vi "DisposeCore.vi"(8 "error in (no error)":errorcluster, 11 "ProductA":refnum<class "ProductA.lvclass">) -> (0 "error out":errorcluster, 3 "ProductA":refnum<class "ProductA.lvclass">)   [LabVIEW 2020, in "FactoryMethod.lvlib" / "FactoryMethodLazyEvaluation.lvlib" / "ProductA.lvclass"]
uses:
  ProductA.lvclass
  Private/TypeDef/privateDataDVR.ctl
  Private/TypeDef/privateData.ctl
  ProductA.lvclass/ProductA.ctl
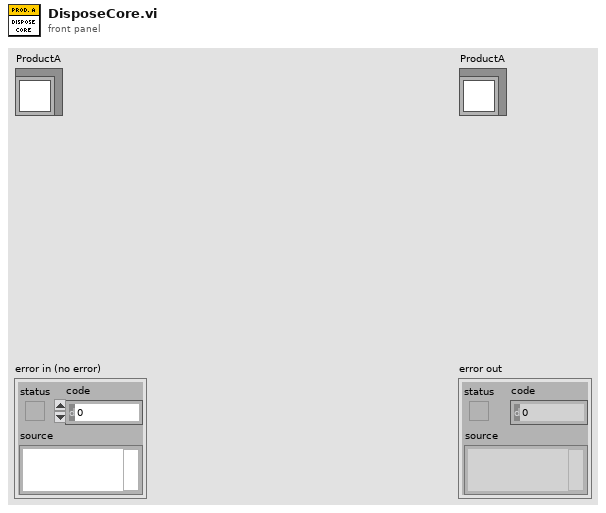
[diagram p1: front panel]
types:
  T1 = typedef "FactoryMethod.lvlib/FactoryMethodLazyEvaluation.lvlib/ProductA.lvclass/privateDataDVR.ctl" = refnum<data-value>
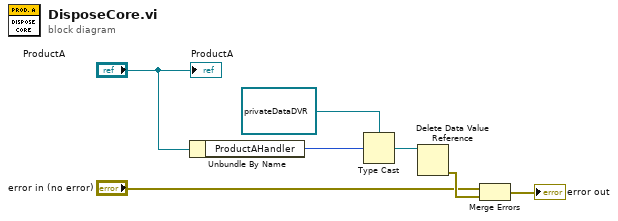
[diagram p0: block diagram]
diagram:
  n1 = Unbundle By Name("ProductA") -> ("ProductAHandler"=w7:u32)
  n2 = Type Cast(type=T1 refnum ("privateDataDVR"), x=w7) -> (*(type *) &x=w5:T1)
  n3 = Delete Data Value Reference(data value reference=w5) -> (error out=w3:errorcluster)  [unwired: 1 in, 1 out]
  n4 = Merge Errors("error in (no error)", w3) -> (→"error out":errorcluster)
  "ProductA" <- "ProductA"
